vi "simulation in arm.vi"() -> ()   [LabVIEW 2024]
uses:
  ME121-25-main/ME121-25-main/LabVIEW/SerialVIs/subs/portX.xctl
panel:
  in  "L 2":dbl(slide)=115.0 scale=0.0..200.0
  in  "L 1":dbl(slide)=80.0 scale=0.0..200.0
  out "Angle 2":dbl(knob)=-72.06882847083946 scale=-90.0..90.0
  out "Angle1":dbl(knob)=-45.83837436417874 scale=-90.0..90.0
  out "resulting string":string
  out "text":string
  out "2D Picture":picture
  out "Cluster":cluster{dbl, dbl}
  in  "file (use dialog)":path
  in  "portX":refnum<visa-resource-name>(xcontrol)
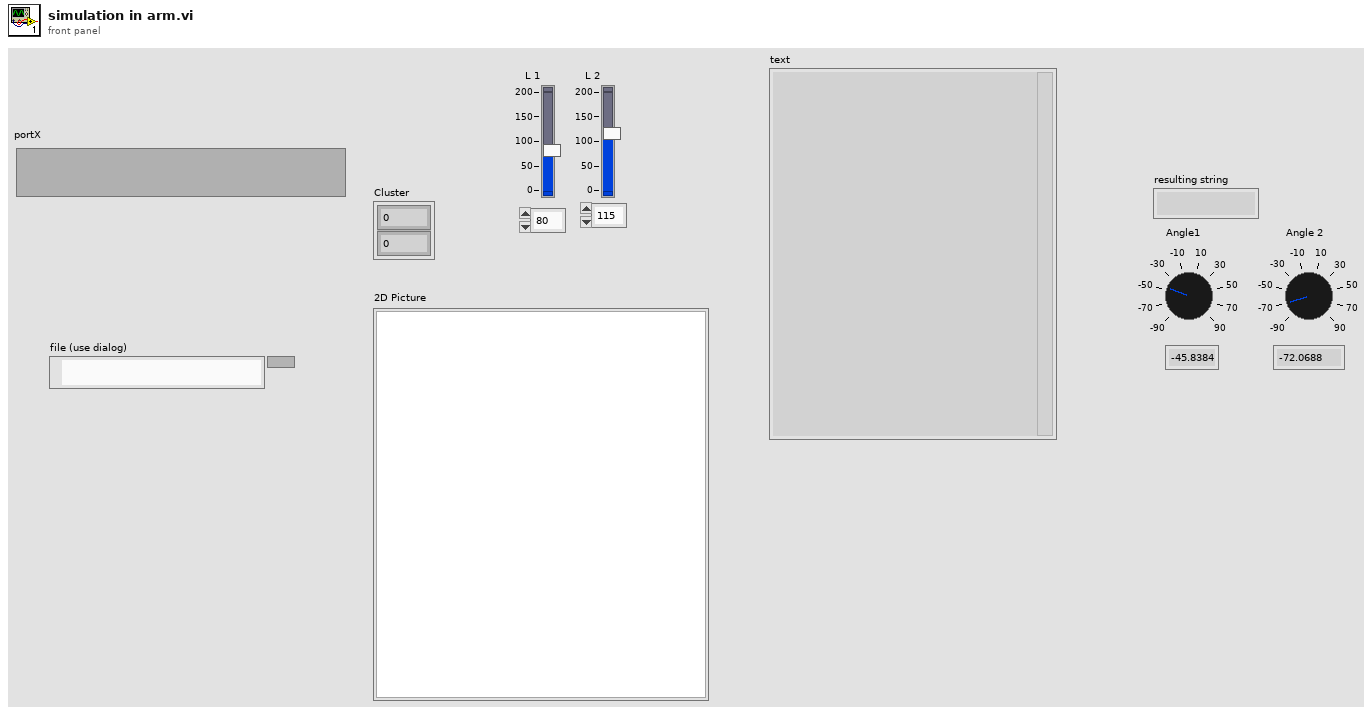
[diagram p1: front panel]
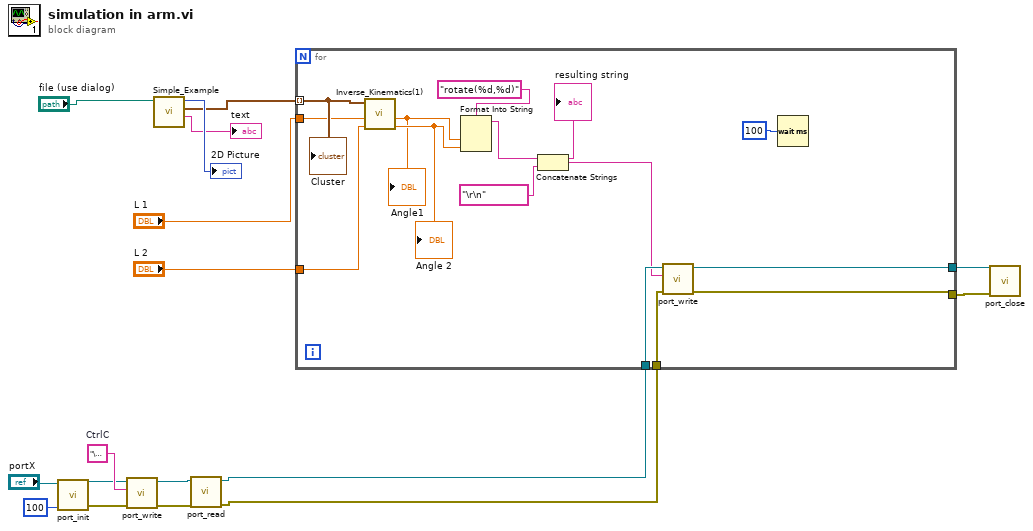
[diagram p0: block diagram]
diagram:
  w17 = "\u0003"  # CtrlC
  n1 = call "port_init.vi"("Timeout (ms)"=u32 100, "VISA Refnum in"="portX") -> ("error out"=w15:errorcluster, "VISA Refnum out"=w16:refnum<visa-resource-name>)  [unwired: 8 in]
  n2 = call "port_write.vi"("error in (no error)"=w15, "write buffer"=w17, "VISA Refnum in"=w16) -> ("error out"=w13:errorcluster, "VISA Refnum out"=w14:refnum<visa-resource-name>)  [unwired: 7 in]
  n3 = call "Simple_Example.vi"("file (use dialog)"="file (use dialog)") -> ("text"=→"text":string, "xy coord"=w4:cluster{"x":dbl, "y":dbl}[], "2D Picture"=→"2D Picture":picture)  [unwired: 8 in]
  n4 = call "port_read.vi"("error in (no error)"=w13, "VISA Refnum in"=w14) -> ("error out"=w7:errorcluster, "VISA Refnum out"=w6:refnum<visa-resource-name>)  [unwired: 7 in, 1 out]
  n5 = for {
    tunnel: w6 -> [w31]
    tunnel: w7 -> [w30]
    tunnel: w4 -> [w29] mode=indexing
    tunnel: [w22] -> w8
    tunnel: [w21] -> w9
    tunnel: "L 1" -> [w19]
    tunnel: "L 2" -> [w18]
    n6 = call "Inverse_Kinematics(1).vi"("L 2"=w18, "L 1"=w19, "end effector"=w29) -> ("Angle 2"=w28:dbl, "Angle1"=w27:dbl)  [unwired: 7 in]
    "Angle1" <- w27
    "Angle 2" <- w28
    n7 = Format Into String(format string="rotate(%d,%d)", w27, w28) -> (resulting string=w25:string)  [unwired: 2 in, 1 out]
    "resulting string" <- w25
    n8 = Concatenate Strings(w25, "\r\n") -> (w23:string)
    n9 = call "port_write.vi"("error in (no error)"=w30, "write buffer"=w23, "VISA Refnum in"=w31) -> ("error out"=w21:errorcluster, "VISA Refnum out"=w22:refnum<visa-resource-name>)  [unwired: 7 in]
    n10 = Wait (ms)(milliseconds to wait=u32 100) -> ()  [unwired: 1 out]
    "Cluster" <- w29
  }
  n11 = call "port_close.vi"("error in (no error)"=w9, "VISA Refnum in"=w8) -> ()  [unwired: 10 in]
